vi "Kelvinox_Parse_PID_to_Number.vi"(1 "PID String":string) -> (0 "PID Number":dbl)   [LabVIEW 2019]
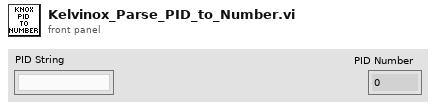
[diagram p1: front panel]
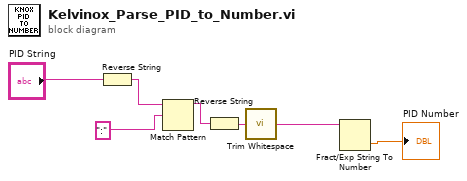
[diagram p0: block diagram]
diagram:
  n1 = Reverse String(1:"PID String") -> (0:w7:string)
  n2 = Match Pattern(string=w7, regular expression=":") -> (before substring=w5:string)  [unwired: 1 in, 3 out]
  n3 = Reverse String(1:w5) -> (0:w3:string)
  n4 = call <vilib>:"Trim Whitespace.vi"("string"=w3) -> ("trimmed string"=w2:string)  [unwired: 1 in]
  n5 = Fract/Exp String To Number(string=w2) -> (number=→"PID Number":dbl)  [unwired: 3 in, 1 out]
